vi "Array-Value Range to Indices.vi"(3 "dx":dbl, 4 "Xmax":dbl, 5 "Xmin":dbl) -> (1 "Length":i32, 2 "Offset":i32)   [LabVIEW 2020]
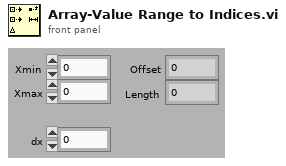
[diagram p1: front panel]
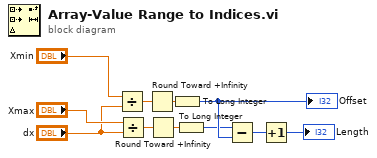
[diagram p0: block diagram]
diagram:
  n1 = Divide(x="Xmin", y="dx") -> (x/y=w1:dbl)
  n2 = Divide(x="Xmax", y="dx") -> (x/y=w2:dbl)
  n3 = Round Toward +Infinity(x=w1) -> (ceil(x): smallest int >= x=w3:dbl)
  n4 = Round Toward +Infinity(x=w2) -> (ceil(x): smallest int >= x=w4:dbl)
  n5 = To Long Integer(number=w3) -> (32bit integer=w9:i32)
  "Offset" <- w9
  n6 = To Long Integer(number=w4) -> (32bit integer=w6:i32)
  n7 = Subtract(x=w6, y=w9) -> (x-y=w7:i32)
  n8 = Increment(x=w7) -> (x+1=→"Length":i32)
